vi "Waveform DRAM element address control.vi"(0 "DRAM address input in":u32, 4 "output valid?":bool) -> (7 "DRAM address output":u32)   [LabVIEW 2015]
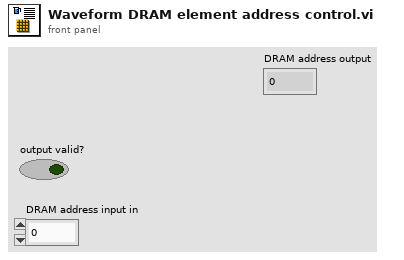
[diagram p1: front panel]
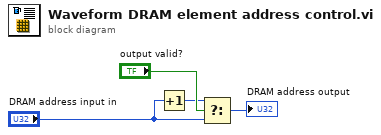
[diagram p0: block diagram]
diagram:
  n1 = Increment(x="DRAM address input in") -> (x+1=w3:u32)
  n2 = Select(t=w3, s="output valid?", f="DRAM address input in") -> (s? t:f=→"DRAM address output":u32)
